vi "BRig_dataBlock_BUR_target.vi"() -> (2 "output_BUR_target":i32)   [LabVIEW 2014]
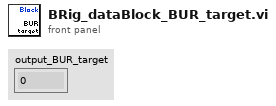
[diagram p1: front panel]
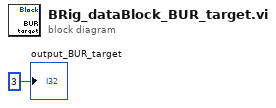
[diagram p0: block diagram]
diagram:
  "output_BUR_target" <- 3 ("output_iBlock")
